vi "InternalDepVI.vi"(11 "Numeric":dbl) -> (3 "Numeric 2":dbl)   [LabVIEW 2017, in "InternalDep.lvlib"]
uses:
  InternalDep.lvlib
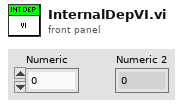
[diagram p1: front panel]
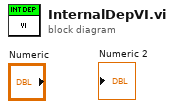
[diagram p0: block diagram]
diagram:
